vi "Actor Core.vi"(8 "error in":errorcluster, 11 "Software Lock-in in":refnum<class "Software Lock-in.lvclass">) -> (0 "error out":errorcluster, 3 "Actor out":refnum<class "Actor.lvclass">)   [LabVIEW 2015, in "Software Lock-in.lvclass"]
doc: "(<B>Filename</B>: Actor Framework.lvlib:Actor.lvclass:Actor Core.vi)\n\nReceives messages to the actor, reacts to them, and initiates any error handling that may shut the actor down.\n\nDescendant classes may override this VI to append parallel tasks for the actor to complete while it handles messages. Overrides use the Call Parent Method node."
uses:
  Software Lock-in.lvclass
  <vilib>/ActorFramework/Actor/Actor.lvclass
  Mag Lab Hardware.lvclass
  Mag Lab Error Handler/Mag Lab Error Handler.lvclass
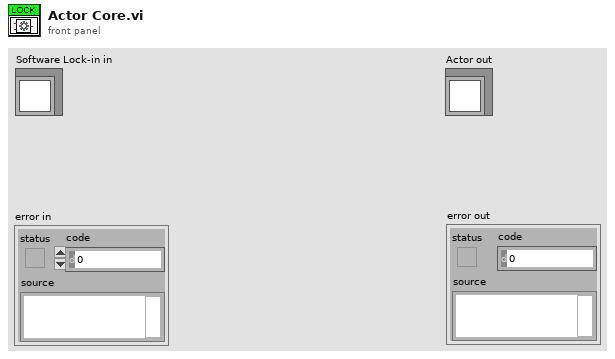
[diagram p1: front panel]
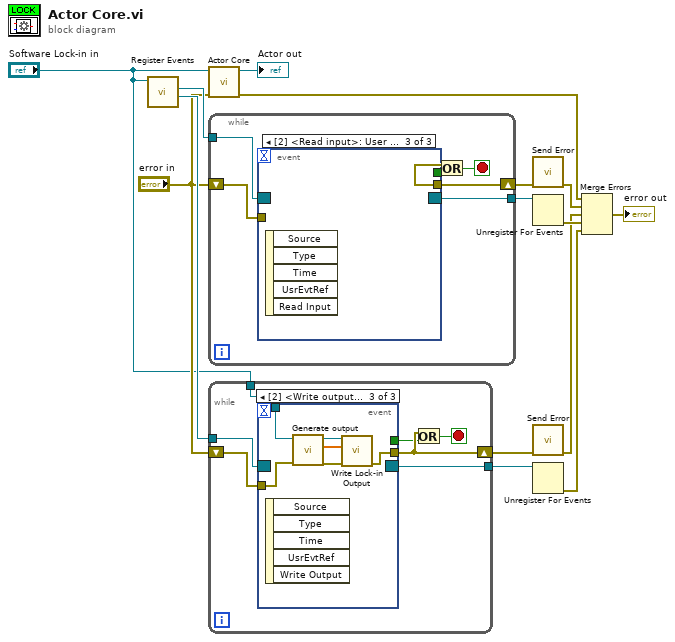
[diagram p0: block diagram]
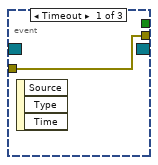
[diagram p2: hidden frame]
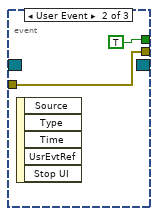
[diagram p3: hidden frame]
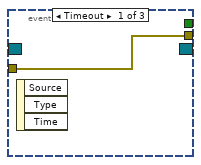
[diagram p4: hidden frame]
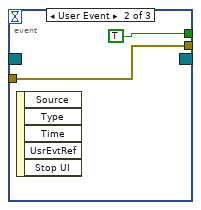
[diagram p5: hidden frame]
diagram:
  n1 = call-dynamic "Register Events.vi"("Software Lock-in in"="Software Lock-in in") -> ("Output Events"=w12:refnum<event-registration>, "Input Events"=w14:refnum<event-registration>)  [unwired: 7 in, 2 out]
  n2 = call-parent "Actor Core.vi"("error in"="error in", "Mag Lab Measure Base in"="Software Lock-in in") -> ("error out"=w10:errorcluster, "Actor out"=→"Actor out":refnum<class "Actor.lvclass">)  [unwired: 8 in]
  n3 = while {
    tunnel: w14 -> [w21]
    tunnel: [w20] -> w13
    shift-right: [w17] -> w3
    shift-left: "error in" -> [w19]
    stop <- w16 stop-if-true
    n4 = event shown="[2] <Read input>: User Event" {
      selector: w21 -> [_ _ _]
      dyn-events: [_ _ _] -> w20
      timeout: _ -> [_ _ _]
      tunnel: [_ TRUE _] -> w18
      tunnel: w19 -> [w22 w23 _]
      tunnel: [w22 w23 _] -> w17
      event Timeout {
        n5 = event-data() -> ()  [unwired: 1 in, 3 out]
      }
      event User Event {
        n6 = event-data() -> ()  [unwired: 1 in, 5 out]
      }
      event User Event {
        n7 = event-data() -> ()  [unwired: 1 in, 5 out]
      }
    }
    n8 = Or(x=w17, y=w18) -> (x .or. y?=w16:bool)
  }
  n9 = while {
    tunnel: w12 -> [w31]
    tunnel: [w30] -> w7
    shift-right: [w28] -> w5
    shift-left: "error in" -> [w29]
    tunnel: "Software Lock-in in" -> [w25]
    stop <- w26 stop-if-true
    n10 = event shown="[2] <Write output>: User Event" {
      selector: w31 -> [_ _ _]
      dyn-events: [_ _ _] -> w30
      timeout: _ -> [_ _ _]
      tunnel: [_ TRUE _] -> w27
      tunnel: w29 -> [w32 w33 w39]
      tunnel: [w32 w33 w36] -> w28
      tunnel: w25 -> [_ _ w40]
      event Timeout {
        n11 = event-data() -> ()  [unwired: 1 in, 3 out]
      }
      event User Event {
        n12 = event-data() -> ()  [unwired: 1 in, 5 out]
      }
      event User Event {
        n13 = event-data() -> ()  [unwired: 1 in, 5 out]
        n14 = call-dynamic "Generate output.vi"("error in (no error)"=w39, "Software Lock-in in"=w40) -> ("error out"=w38:errorcluster, "Sine wave"=w35:dbl[], "Software Lock-in out"=w37:refnum<class "Software Lock-in.lvclass">)  [unwired: 7 in]
        n15 = call-dynamic "Write Lock-in Output.vi"("error in (no error)"=w38, "Output data"=w35, "Software Lock-in in"=w37) -> ("error out"=w36:errorcluster)  [unwired: 7 in, 1 out]
      }
    }
    n16 = Or(x=w28, y=w27) -> (x .or. y?=w26:bool)
  }
  n17 = call "Send Error.vi"("error in (no error)"=w3) -> ("error out"=w2:errorcluster)  [unwired: 9 in, 1 out]
  n18 = Unregister For Events(event registration refnum=w13) -> (error out=w8:errorcluster)  [unwired: 1 in]
  n19 = call "Send Error.vi"("error in (no error)"=w5) -> ("error out"=w4:errorcluster)  [unwired: 9 in, 1 out]
  n20 = Unregister For Events(event registration refnum=w7) -> (error out=w6:errorcluster)  [unwired: 1 in]
  n21 = Merge Errors(w10, w2, w4, w8, w6) -> (→"error out":errorcluster)
